vi "Sensitivity (2).vi"(9 "Power (z)":dbl min=0.0 step=0.1, 10 "Sensitivity (a)":dbl step=0.1, 11 "Input":dbl(slide) scale=-1.0..1.0) -> (3 "Output":dbl(slide) scale=-1.0..1.0)   [LabVIEW 2016]
panel:
  out "XY Graph":cluster{dbl[], dbl[]}(graph)
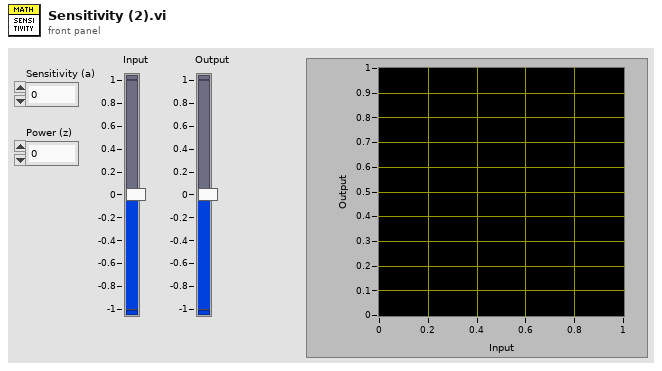
[diagram p1: front panel]
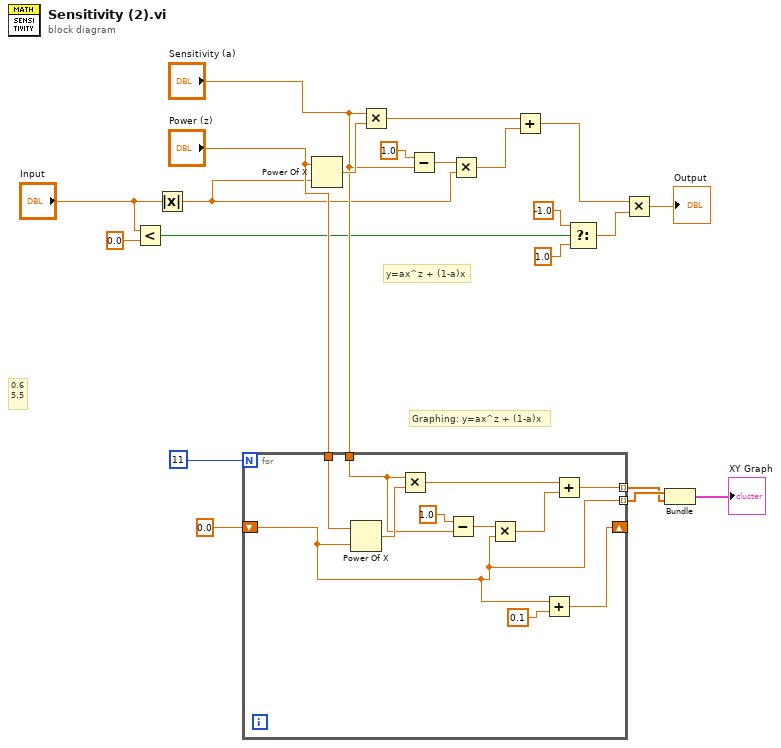
[diagram p0: block diagram]
diagram:
  # "Graphing: y=ax^z + (1-a)x"
  # "0.6\n5.5"
  # "y=ax^z + (1-a)x"
  n1 = Less?(x="Input", y=0.0) -> (x < y?=w8:bool)
  n2 = Absolute Value(x="Input") -> (abs(x)=w6:dbl)
  n3 = for {
    N: 11 -> [_]
    shift-right: [w24] -> _
    shift-left: 0.0 -> [w22]
    tunnel: "Sensitivity (a)" -> [w27]
    tunnel: "Power (z)" -> [w26]
    tunnel: [w23] -> w2 mode=indexing
    tunnel: [w22] -> w3 mode=indexing
    n4 = Power Of X(1:w22, 2:w26) -> (0:w32:dbl)
    n5 = Multiply(x=w27, y=w32) -> (x*y=w31:dbl)
    n6 = Subtract(x=1.0, y=w27) -> (x-y=w29:dbl)
    n7 = Multiply(x=w29, y=w22) -> (x*y=w28:dbl)
    n8 = Add(x=w22, y=0.1) -> (x+y=w24:dbl)
    n9 = Add(x=w31, y=w28) -> (x+y=w23:dbl)
  }
  n10 = Power Of X(1:w6, 2:"Power (z)") -> (0:w21:dbl)
  n11 = Multiply(x="Sensitivity (a)", y=w21) -> (x*y=w20:dbl)
  n12 = Subtract(x=1.0, y="Sensitivity (a)") -> (x-y=w18:dbl)
  n13 = Multiply(x=w18, y=w6) -> (x*y=w17:dbl)
  n14 = Add(x=w20, y=w17) -> (x+y=w13:dbl)
  n15 = Select(t=-1.0, s=w8, f=1.0) -> (s? t:f=w11:dbl)
  n16 = Multiply(x=w13, y=w11) -> (x*y=→"Output":dbl)
  n17 = Bundle(w3, w2) -> (→"XY Graph":cluster{dbl[], dbl[]})  [unwired: 1 in]
